vi "LEBITVacuum.PubAmbientMeasurments.vi"(0 "i ref in":refnum<vi>, 2 "i attribute in":T1={"setValuePLC"=[], "nickNames"=[], "setValuePLCServiceID"=[], "monValuePLC"=[], "SetValueServiceID"=[], "MonValueServiceID"=[], "SetValue"=[], "AllPLCValues"=[], "CondSpecial2DArray"=[], "CondSpecialIndex"=[], "ReasonForLocking"="", "ReasonForLockingID"=0, "enableValuePLC"=[], "OverwriteCloseSafetyPLC"=[], "OverwriteOpenSafetyPLC"=[], "OverwriteCloseSafetyPLCServiceID"=[], "OverwriteOpenSafetyPLCServiceID"=[], "MKS Address Array"=[], "MKS MeasurementServiceID"=[], "MKS Measurement"=[], "CRYO Measurement"=[], "CRYO MeasurementServiceID"=[], "Special"=[], "Start Date"="", "MKS VISA resource"="COM13", "CRYO VISA resource"="COM13"}, 5 "error in":errorcluster) -> (14 "i ref out":refnum<vi>, 16 "i attribute out":T1={"setValuePLC"=[], "nickNames"=[], "setValuePLCServiceID"=[], "monValuePLC"=[], "SetValueServiceID"=[], "MonValueServiceID"=[], "SetValue"=[], "AllPLCValues"=[], "CondSpecial2DArray"=[], "CondSpecialIndex"=[], "ReasonForLocking"="", "ReasonForLockingID"=0, "enableValuePLC"=[], "OverwriteCloseSafetyPLC"=[], "OverwriteOpenSafetyPLC"=[], "OverwriteCloseSafetyPLCServiceID"=[], "OverwriteOpenSafetyPLCServiceID"=[], "MKS Address Array"=[], "MKS MeasurementServiceID"=[], "MKS Measurement"=[], "CRYO Measurement"=[], "CRYO MeasurementServiceID"=[], "Special"=[], "Start Date"="", "MKS VISA resource"="COM13", "CRYO VISA resource"="COM13"}, 17 "MKS MeasurementServiceID":i32[](array[numeric]), 18 "CRYO MeasurementServiceID":i32[](array[numeric]), 19 "error out":errorcluster)   [LabVIEW 2014, in "LEBITVacuum.lvlib"]
uses:
  LEBITVacuum.lvlib
  LEBITVacuum.i attribute.ctl
  CSlibraries/UtilityLib/UtilityLib.valueStatus.ctl
  CSlibraries/UtilityLib/UtilityLib.lvlib
  CSCore/CSSystem/CoreLib/CoreLib.lvlib
  CSlibraries-extern/DimLVEvent/LVDimInterface/LVDimInterface.lvlib
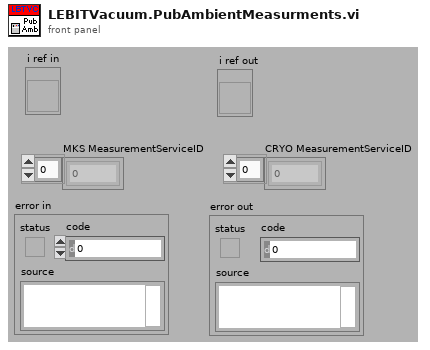
[diagram p1: front panel]
types:
  T1 = typedef "LEBITVacuum.lvlib/LEBITVacuum.i attribute.ctl" = cluster{"setValuePLC":string[], "nickNames":string[], "setValuePLCServiceID":i32[], "monValuePLC":string[], "SetValueServiceID":i32[], "MonValueServiceID":i32[], "SetValue":i16[], "AllPLCValues":string[], "CondSpecial2DArray":string[][], "CondSpecialIndex":i32[], "ReasonForLocking":string, "ReasonForLockingID":i32, "enableValuePLC":string[], "OverwriteCloseSafetyPLC":string[], "OverwriteOpenSafetyPLC":string[], "OverwriteCloseSafetyPLCServiceID":i32[], "OverwriteOpenSafetyPLCServiceID":i32[], "MKS Address Array":i32[][], "MKS MeasurementServiceID":i32[], "MKS Measurement":string[], "CRYO Measurement":string[][], "CRYO MeasurementServiceID":i32[], "Special":string[], "Start Date":string, "MKS VISA resource":refnum<visa-resource-name>, "CRYO VISA resource":refnum<visa-resource-name>}
  T2 = typedef "UtilityLib.lvlib/UtilityLib.valueStatus.ctl" = enum16{"no info available", "stand by/off", "on", "warning", "alarm/malfunction", "not implemented", "user action required", "important information", "system default", "control default", "indicator default", "button default"}
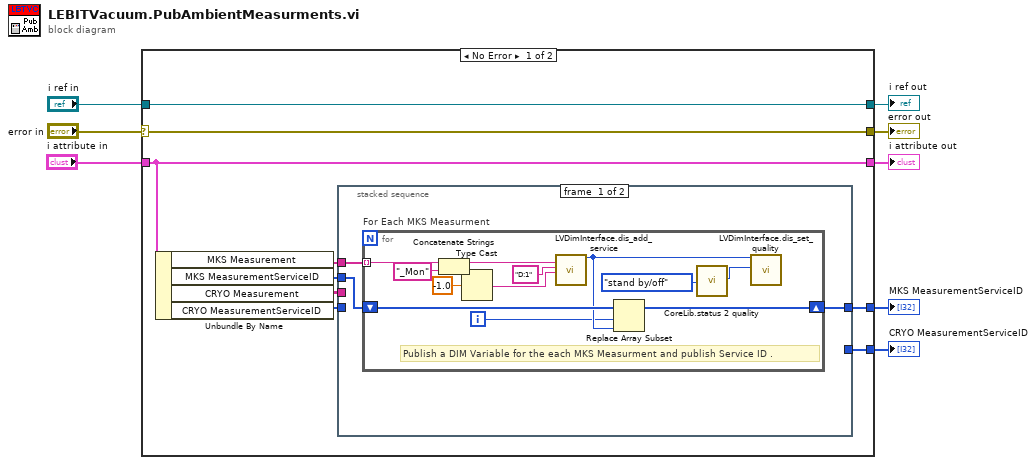
[diagram p0: block diagram]
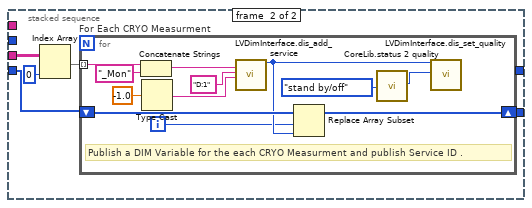
[diagram p2: hidden frame]
diagram:
  n1 = case shown="No Error" "error in" {
    selector: "error in" -> [w17 w51]
    tunnel: "i attribute in" -> [w15 w50]
    tunnel: [w17 w51] -> w8
    tunnel: [w16 w52] -> w7
    tunnel: "i ref in" -> [w16 w52]
    tunnel: [w15 w50] -> w3
    tunnel: [w14 _] -> w2
    tunnel: [w9 _] -> w1
    frame No Error {
      n2 = Unbundle By Name(w15) -> ("MKS Measurement"=w11:string[], "MKS MeasurementServiceID"=w10:i32[], "CRYO Measurement"=w12:string[][], "CRYO MeasurementServiceID"=w13:i32[])
      n3 = stacked-sequence {
        tunnel: [w20 _] -> w14
        tunnel: w13 -> [_ w36]
        tunnel: w12 -> [_ w34]
        tunnel: w11 -> [w19 _]
        tunnel: w10 -> [w18 _]
        tunnel: [_ w35] -> w9
        frame #0 {
          n4 = for "For Each MKS Measurment" {
            tunnel: w19 -> [w22] mode=indexing
            shift-right: [w26] -> w20
            shift-left: w18 -> [w27]
            i -> [w24]
            # "Publish a DIM Variable for the each MKS Measurment and publish Service ID ."
            n5 = Concatenate Strings(w22, "_Mon" ("string")) -> (w21:string)
            n6 = Type Cast(x=-1.0) -> (*(type *) &x=w28:string)  [unwired: 1 in]
            n7 = call "LVDimInterface.dis_add_service.vi"("serviceName"=w21, "typeDescriptor"="D:1", "data"=w28) -> ("my_serviceID"=w25:i32)  [unwired: 15 in, 1 out]
            n8 = Replace Array Subset(array=w27, new element=w25, index=w24) -> (w26:i32[])
            n9 = call "CoreLib.status 2 quality.vi"("valueStatus"=UtilityLib.valueStatus."stand by/off") -> ("quality"=w32:i32)  [unwired: 18 in]
            n10 = call "LVDimInterface.dis_set_quality.vi"("my_serviceID"=w25, "quality"=w32) -> ()  [unwired: 16 in, 2 out]
          }
        }
        frame #1 {
          n11 = Index Array(array=w34, index (col)=0 ("index (row)")) -> (element=w37:string[])  [unwired: 1 in]
          n12 = for "For Each CRYO Measurment" {
            tunnel: w37 -> [w38] mode=indexing
            shift-right: [w43] -> w35
            shift-left: w36 -> [w44]
            i -> [w41]
            # "Publish a DIM Variable for the each CRYO Measurment and publish Service ID ."
            n13 = Concatenate Strings(w38, "_Mon" ("string")) -> (w39:string)
            n14 = Type Cast(x=-1.0) -> (*(type *) &x=w45:string)  [unwired: 1 in]
            n15 = call "LVDimInterface.dis_add_service.vi"("serviceName"=w39, "typeDescriptor"="D:1", "data"=w45) -> ("my_serviceID"=w42:i32)  [unwired: 15 in, 1 out]
            n16 = Replace Array Subset(array=w44, new element=w42, index=w41) -> (w43:i32[])
            n17 = call "CoreLib.status 2 quality.vi"("valueStatus"=UtilityLib.valueStatus."stand by/off") -> ("quality"=w49:i32)  [unwired: 18 in]
            n18 = call "LVDimInterface.dis_set_quality.vi"("my_serviceID"=w42, "quality"=w49) -> ()  [unwired: 16 in, 2 out]
          }
        }
      }
    }
    frame Error {
    }
  }
  "error out" <- w8
  "i ref out" <- w7
  "i attribute out" <- w3
  "MKS MeasurementServiceID" <- w2
  "CRYO MeasurementServiceID" <- w1
